vi "RSZVB Load And Interchange Single Ended Port Circuit Model Data.vi"(6 "File Name (\"\")":string, 7 "Physical Port Number (1)":i32=1, 8 "error in (no error)":errorcluster {"code" format="%.0x"}, 9 "Function Type (Deembedding)":i32(ring) items=["Deembedding", "Embedding"], 10 "Channel (1)":i32=1, 11 "VISA session":refnum<visa-resource-name>) -> (0 "error out":errorcluster {"code" format="%.0x"}, 3 "dup VISA session":refnum<visa-resource-name>)   [LabVIEW 2011]
doc: "This VI loads data from a specified two-port (*.sp2) Touchstone file defining the characteristics of the current embedded/deembedded single ended port circuit model. The single ended port circuit model involving file import (FIMPort) must be selected before using this VI. \n\nRemote-control command(s):\nMMEMory:LOAD:VNETworks<Ch>:SENDed:EMBedding<Ph_pt> '<file_name>',IPORt \nMMEMory:LOAD:VNETworks<Ch>:SENDed:DEEMbedding<Ph_pt> '<file_name>',IPORt"
uses:
  _utility/RSZVB Global Data.vi
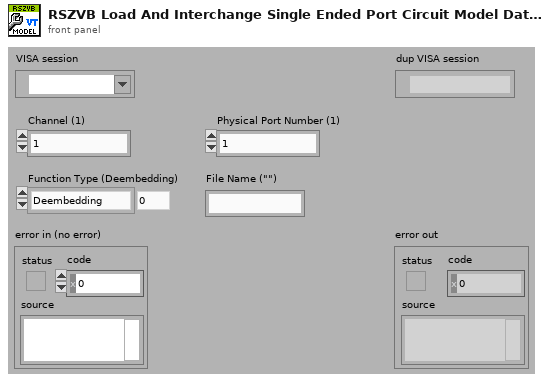
[diagram p1: front panel]
types:
  T1 = cluster{"Error Checking (T: On)":bool, "Installed Options":string[], "Data Valid?":bool, "Ports":i32, "Model":string[], "Option Checking (T: On)":bool}[]
  T2 = cluster{"Error Checking (T: On)":bool, "Installed Options":string[], "Data Valid?":bool, "Ports":i32, "Model":string[], "Option Checking (T: On)":bool}
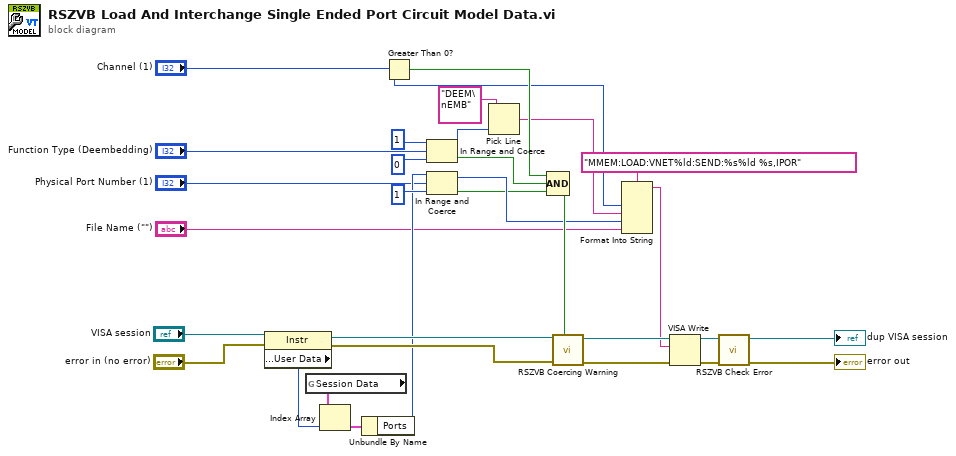
[diagram p0: block diagram]
diagram:
  n1 = property class="Instr"(reference="VISA session", error in="error in (no error)") -> (reference out=w21:refnum<visa-resource-name>, error out=w22:errorcluster, "General Settings:User Data"=w25:u32)
  n2 = global read "RSZVB Global Data.vi" "Session Data"() -> (w24:T1)
  n3 = Index Array(array=w24, index=w25) -> (element=w23:T2)
  n4 = Unbundle By Name(w23) -> ("Ports"=w9:i32)
  n5 = Greater Than 0?(x="Channel (1)") -> (x > 0?=w18:bool)
  n6 = In Range and Coerce(upper limit=1 ("lower limit"), x="Function Type (Deembedding)", lower limit=0) -> (coerced(x)=w12:i32, In Range?=w15:bool)
  n7 = In Range and Coerce(upper limit=w9, x="Physical Port Number (1)", lower limit=1) -> (coerced(x)=w14:i32, In Range?=w10:bool)
  n8 = Pick Line(multi-line string="DEEM\nEMB", line index=w12) -> (output string=w11:string)  [unwired: 1 in]
  n9 = Compound Arithmetic op=AND(w18, w15, w10) -> (w17:bool)
  n10 = call "RSZVB Coercing Warning.vi"("In Range?"=w17, "error in (no error)"=w22, "VISA session"=w21) -> ("error out"=w30:errorcluster, "dup VISA session"=w31:refnum<visa-resource-name>)  [unwired: 7 in]
  n11 = Format Into String(format string="MMEM:LOAD:VNET%ld:SEND:%s%ld %s,IPOR", "Channel (1)", w11, w14, "File Name (\"\")") -> (resulting string=w26:string)  [unwired: 2 in, 1 out]
  n12 = VISA Write(VISA resource name=w31, write buffer=w26, error in (no error)=w30) -> (VISA resource name out=w28:refnum<visa-resource-name>, error out=w29:errorcluster)  [unwired: 1 out]
  n13 = call "RSZVB Check Error.vi"("error in (no error)"=w29, "VISA session"=w28) -> ("error out"=→"error out":errorcluster, "dup VISA session"=→"dup VISA session":refnum<visa-resource-name>)  [unwired: 8 in]
